vi "Read settings id.vi"(8 "error in (no error)":errorcluster, 11 "DSFGroup in":refnum<class "DSFGroup.lvclass">) -> (0 "error out":errorcluster, 2 "settings id":string, 3 "DSFGroup out":refnum<class "DSFGroup.lvclass">)   [LabVIEW 2017, in "DSFGroup.lvclass"]
uses:
  DSFGroup.lvclass
  DSFGroup.lvclass/DSFGroup.ctl
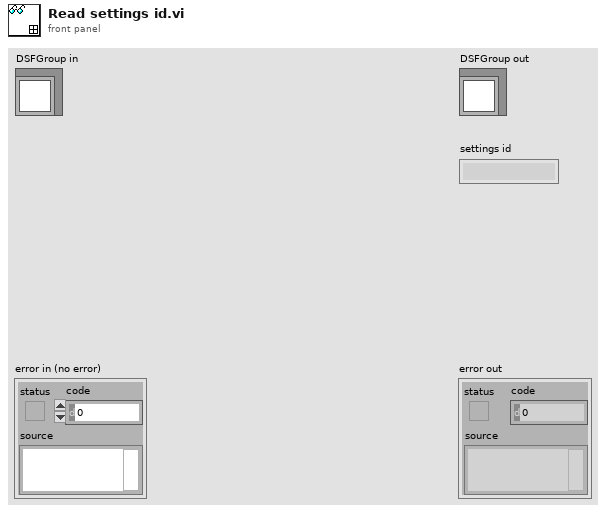
[diagram p1: front panel]
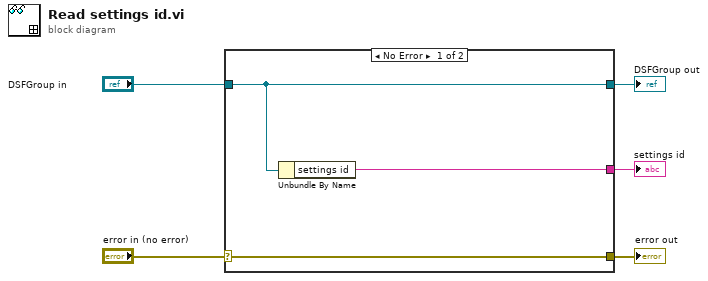
[diagram p0: block diagram]
diagram:
  n1 = case shown="No Error" "error in (no error)" {
    selector: "error in (no error)" -> [w8 w9]
    tunnel: [w8 w9] -> w4
    tunnel: [w7 w10] -> w2
    tunnel: "DSFGroup in" -> [w7 w10]
    tunnel: [w6 _] -> w1
    frame No Error {
      n2 = Unbundle By Name(w7) -> ("settings id"=w6:string)
    }
    frame Error {
    }
  }
  "error out" <- w4
  "DSFGroup out" <- w2
  "settings id" <- w1
